vi "PV Set decimal separator.vi"() -> (0 "decimal separator":string)   [LabVIEW 2024, in "Pfeiffer Vacuum.lvlib"]
uses:
  <instrlib>/Pfeiffer Vacuum/Pfeiffer Vacuum.lvlib
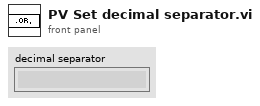
[diagram p1: front panel]
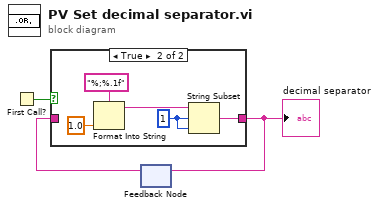
[diagram p0: block diagram]
diagram:
  n1 = First Call?() -> (First Call?: T/F=w1:bool)
  n2 = feedback #1() -> (w2:string)  [unwired: 1 in]
  n3 = case shown="True" w1 {
    tunnel: [w4 w7] -> w3
    tunnel: w2 -> [w4 _]
    frame False {
    }
    frame True {
      w5 = 1 ("offset (0)")
      n4 = Format Into String(format string="%;%.1f", 1.0 ("input 1")) -> (resulting string=w6:string)  [unwired: 2 in, 1 out]
      n5 = String Subset(string=w6, offset (0)=w5, length (rest)=w5) -> (substring=w7:string)
    }
  }
  "decimal separator" <- w3
  n6 = feedback-in #1(w3) -> ()
